vi "get_single_acq.vi"(8 "error in (no error)":errorcluster, 11 "ibsen in":refnum<class "ibsen.lvclass">) -> (0 "error out":errorcluster, 1 "trigger":dbl[][](array[numeric]), 2 "raw data":i32[][][](array[numeric]), 3 "ibsen out":refnum<class "ibsen.lvclass">)   [LabVIEW 2019, in "ibsen.lvlib" / "ibsen.lvclass"]
uses:
  ibsen.lvclass
  D:/github/TransientAbsorptionDAQ.lv/_camera/_camera.lvlibp/_cameraClass/_camera.lvclass
  ibsen.lvclass/ibsen.ctl
  _camera/_camera.lvlibp/_cameraClass/Read background.vi
panel:
  out "Waveform Graph":i32[](graph)
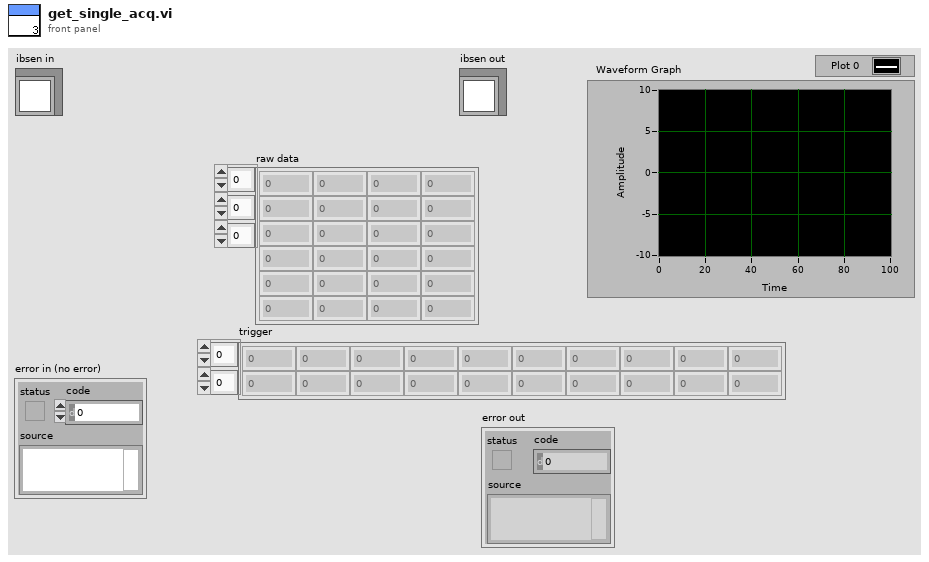
[diagram p1: front panel]
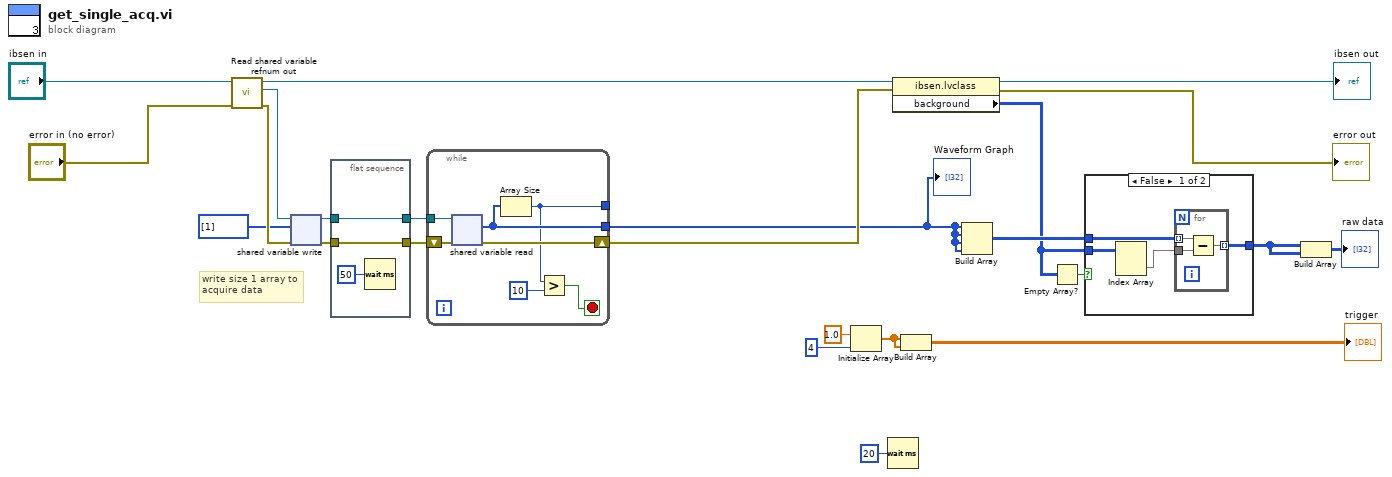
[diagram p0: block diagram]
diagram:
  # "write size 1 array to\nacquire data"
  n1 = call "Read shared variable refnum out.vi"("error in (no error)"="error in (no error)", "ibsen in"="ibsen in") -> ("error out"=w7:errorcluster, "shared variable refnum out"=w8:refnum<k21>, "ibsen out"=w10:refnum<class "ibsen.lvclass">)  [unwired: 7 in]
  n2 = shared-variable-write(w8, w7, i32[] [1] ("data in")) -> (w4:refnum<k21>, w2:errorcluster)
  n3 = flat-sequence {
    tunnel: [w26] -> w5
    tunnel: w4 -> [w26]
    tunnel: [w25] -> w3
    tunnel: w2 -> [w25]
    frame #0 {
      n4 = Wait (ms)(milliseconds to wait=u32 50) -> ()  [unwired: 1 out]
    }
  }
  n5 = while {
    tunnel: [w33] -> w1
    tunnel: [w30] -> _
    tunnel: w5 -> [w32]
    shift-right: [w34] -> w9
    shift-left: w3 -> [w31]
    stop <- w28 stop-if-true
    n6 = shared-variable-read(w32, w31) -> (w34:errorcluster, w33:i32[])  [unwired: 2 out]
    n7 = Array Size(array=w33) -> (size(s)=w30:i32)
    n8 = Greater?(x=w30, y=10) -> (0:w28:bool)
  }
  "Waveform Graph" <- w1
  n9 = Initialize Array(1.0 ("element"), 4 ("dimension size")) -> (w20:dbl[])
  n10 = Wait (ms)(milliseconds to wait=u32 20) -> ()  [unwired: 1 out]
  n11 = property class="ibsen.lvclass"(reference=w10, error in=w9) -> (reference out=→"ibsen out":refnum<class "ibsen.lvclass">, error out=→"error out":errorcluster, "background"=w15:i32[][])
  n12 = Build Array(w20, w20) -> (→"trigger":dbl[][])
  n13 = Build Array(w1, w1, w1, w1) -> (w17:i32[][])
  n14 = Empty Array?(array=w15) -> (empty?=w18:bool)
  n15 = case shown="False" w18 {
    tunnel: w17 -> [w38 w42]
    tunnel: [w37 w42] -> w16
    tunnel: w15 -> [w36 _]
    frame False {
      n16 = Index Array(array=w36) -> (element=w35:i32[])  [unwired: 2 in]
      n17 = for {
        tunnel: w38 -> [w41] mode=indexing
        tunnel: [w40] -> w37 mode=indexing
        tunnel: w35 -> [w39]
        n18 = Subtract(x=w41, y=w39) -> (x-y=w40:i32[])
      }
    }
    frame True {
    }
  }
  n19 = Build Array(w16, w16) -> (→"raw data":i32[][][])
